vi "Acquisition Core.vi"(6 "Acquired z-plane index":i32, 8 "error in":errorcluster, 9 "AOL_Globals":T5={"Imaging Protocol"=enum."AOL Z-Stack", "Number of POI"=0, "Number of Miniscans"=0, "Number of Trials"=0, "Number of Cycles "=0, "# Averaged Frames"=0, "Laser power (%)"=0, "Pockels"=0.0, "Acquisition Length (sec)"=0.0, "Fill time (us)"=0.0, "POI Dwell time (us)"=0.0, "Miniscan Dwell time per pixel (us)"=0.0, "PMT 1"=0.0, "PMT 2"=0.0, "Back Apperture"=200.0, "Frame Size"=0, "Center Frequency"=0.0, "Field of View"=0.0, "DwellTime (us)"=0.0, "Wavelength (nm)"=0.0, "Zoom"=0.0, "AOL Z"=0.0, "AOL Mode"=enum."Raster", "GridXY"=0.0, "GridZ"=0.0, "TriggerPeriod (sec)"=0.0, "Number of Pixels in Miniscan"=0, "Experiment folder path"=path "", "X centre"=0.0, "Y centre"=0.0, "Angle (degrees)"=0.0, "Plane Mode"=0, "Threshold"=[], "Regenerate Chirps"=FALSE, "Rectangle ROI length (pixels)"=0, "Rectangle ROI height (pixels)"=0, "AOD fill"=0, "Samples Wait after Trigger"=0, "StartUp Delay"=0, "Slip Cycle"=163840, "Add Cycle"=FALSE} {"Plane Mode" items=["XY Plane"]; "Frame Size" items=["100X100"=100, "128X128"=128, "200X200"=200, "256X256"=256, "512X512"=512, "1024x1024"=1024, "2048x2048"=2048]; "Back Apperture" format="%#.6g"; "Pockels" format="%#.6g"; "PMT 2" format="%#.6g"; "PMT 1" format="%#.6g"; "Angle (degrees)" format="%#.6g"; "POI Dwell time (us)" format="%#.6g"}, 11 "Logging queue in":T8) -> (0 "error out":errorcluster, 1 "Logging queue element":T1={"Imaging Protocol"=enum."Live Imaging", "Number of Trials"=0, "Frame Size"=512, "# Averaged frames"=0, "Dwell time (us)"=0.0, "Index of Z-plane"=0, "Timelapse?"=FALSE, "Logging process is active"=FALSE, "Speed logging enabled"=FALSE, "tdms file ref"=refnum, "path"=path "", "Trial Number"=0, "Expected # points acquired"=FALSE, "Manually stopped"=FALSE, "Ch0 data"=[], "Ch1 data"=[], "Last trial"=FALSE, "Points acquired"={"Ch0 last trial"=0, "Ch1 last trial"=0, "All trials"=0}} {"Frame Size" items=["100X100"=100, "128X128"=128, "200X200"=200, "256X256"=256, "512X512"=512, "1024x1024"=1024, "2048x2048"=2048]; "Dwell time (us)" format="%#.6g"})   [LabVIEW 2013]
uses:
  Typedefs/Data queue ref.ctl
  Typedefs/Logging queue element.ctl
  Typedefs/Imaging Protocols enum.ctl
  Typedefs/Frame Size.ctl
  Typedefs/Acquired points count.ctl
  Typedefs/Controls/AOL_Globals.ctl
  Typedefs/AOL modes.ctl
  Typedefs/Plane Mode.ctl
  Typedefs/HW config states enum.ctl
  Video Rec Signaling/typedefs/Functions enum.ctl
  Global Variables/General Globals.vi
panel:
  out "subVI exec time":u32
  out "VI exec time":u32
  out "Elements Remaining in FIFO":u32
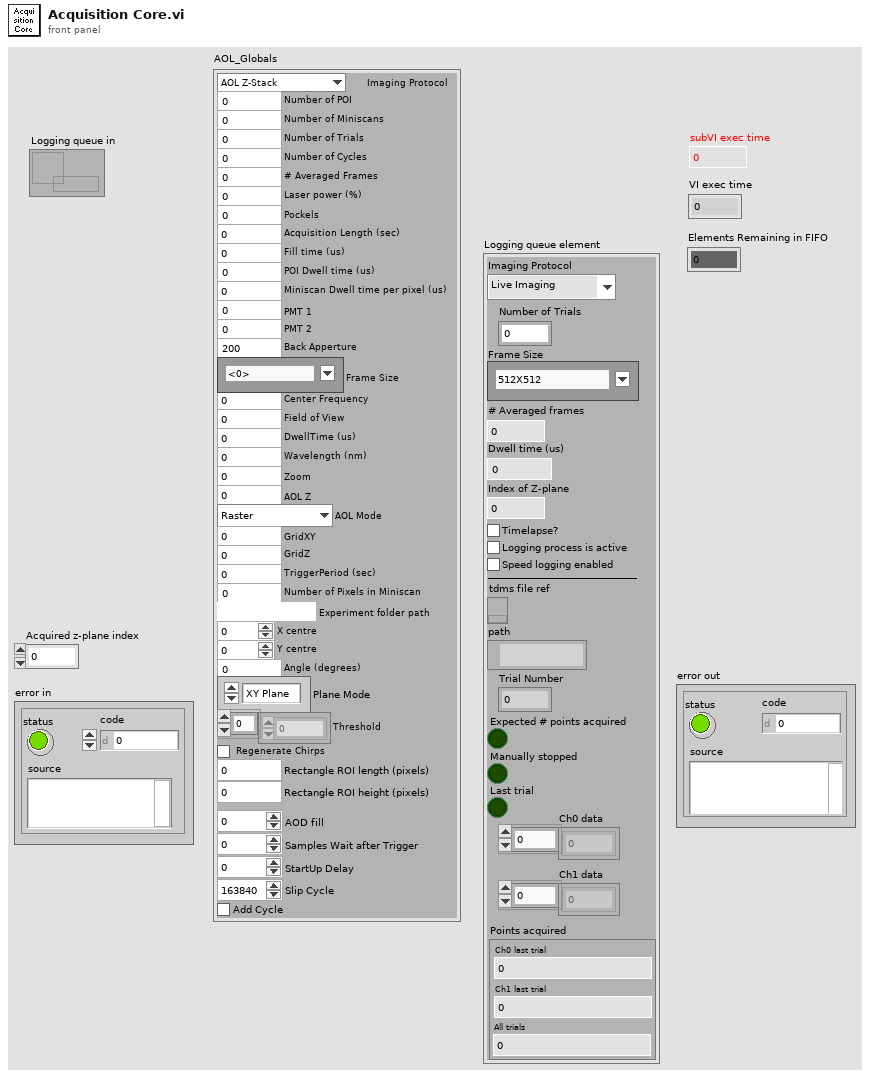
[diagram p1: front panel]
types:
  T1 = typedef "Logging queue element.ctl" = cluster{"Imaging Protocol":T2, "Number of Trials":u16, "Frame Size":T3, "# Averaged frames":u16, "Dwell time (us)":dbl, "Index of Z-plane":i32, "Timelapse?":bool, "Logging process is active":bool, "Speed logging enabled":bool, "tdms file ref":refnum<k34>, "path":path, "Trial Number":i32, "Expected # points acquired":bool, "Manually stopped":bool, "Ch0 data":u32[], "Ch1 data":u32[], "Last trial":bool, "Points acquired":T4}
  T2 = typedef "Imaging Protocols enum.ctl" = enum16{"AOL Z-Stack", "Motor Z Stack", "Functional Acquisition", "Single Plane Acquisition", "Volume Acquisition", "Live Imaging", "Live Plane Imaging", "Live Volume Imaging"}
  T3 = typedef "Frame Size.ctl" = u16
  T4 = typedef "Acquired points count.ctl" = cluster{"Ch0 last trial":u64, "Ch1 last trial":u64, "All trials":u64}
  T5 = typedef "AOL_Globals.ctl" = cluster{"Imaging Protocol":T2, "Number of POI":u16, "Number of Miniscans":u16, "Number of Trials":u16, "Number of Cycles ":u64, "# Averaged Frames":u16, "Laser power (%)":u8, "Pockels":dbl, "Acquisition Length (sec)":dbl, "Fill time (us)":dbl, "POI Dwell time (us)":dbl, "Miniscan Dwell time per pixel (us)":dbl, "PMT 1":dbl, "PMT 2":dbl, "Back Apperture":dbl, "Frame Size":T3, "Center Frequency":dbl, "Field of View":dbl, "DwellTime (us)":dbl, "Wavelength (nm)":dbl, "Zoom":dbl, "AOL Z":dbl, "AOL Mode":T6, "GridXY":dbl, "GridZ":dbl, "TriggerPeriod (sec)":dbl, "Number of Pixels in Miniscan":u16, "Experiment folder path":path, "X centre":dbl, "Y centre":dbl, "Angle (degrees)":dbl, "Plane Mode":T7, "Threshold":u16[], "Regenerate Chirps":bool, "Rectangle ROI length (pixels)":u16, "Rectangle ROI height (pixels)":u16, "AOD fill":u16, "Samples Wait after Trigger":u16, "StartUp Delay":i32, "Slip Cycle":u32, "Add Cycle":bool}
  T6 = typedef "AOL modes.ctl" = enum16{"Raster", "Structural", "Pointing", "Mini Scan", "Alignment"}
  T7 = typedef "Plane Mode.ctl" = u16
  T8 = typedef "Data queue ref.ctl" = refnum<queue>
  T9 = typedef "HW config states enum.ctl" = enum16{"Load from file", "Save to file", "Write all", "Read all", "Write XY stage settings", "Write DAQ FPGA settings", "Write Control FPGA settings", "Write Phys Channels", "Clear", "Compare from file"}
  T10 = typedef "Functions enum.ctl" = enum16{"Create", "Start", "Write", "Stop", "Clear"}
  T11 = typedef "Sys Configuration.ctl" = cluster{"XY Stage":T12, "DAQ FPGA":T13, "Control system":T17, "Encoder":T18, "DAQmx Chan":T19, "Computer MAC address":string, "Cam VidRec":T20, "Externalise Triggers":bool, "Laser wavelength (nm)":dbl}
  T12 = typedef "XY Stage config cluster.ctl" = cluster{"COM port":refnum<visa-resource-name>, "XY stage available":bool}
  T13 = typedef "DAQ FPGA config cluster.ctl" = cluster{"Ref":T14, "Target":T15, "Clock Freq (MHz) ":dbl, "input card type":T16, "Samples Wait after Trigger":u16, "AOD fill":u16, "StartupDelay":i32, "Slip Cycle (clock cycles)":u32, "Add Cycle":bool}
  T14 = typedef "FPGA Ref.ctl" = refnum<k20>
  T15 = typedef "nirio_resource_hc.ctl" = tag
  T16 = typedef "FPGA input type AC-DC.ctl" = enum16{"AC Card", "DC Card"}
  T17 = typedef "CTRL system config cluster.ctl" = cluster{"Ethernet opened":bool, "Ethernet Port":u32, "Ctrl FPGA available":bool, "Ctrl FPGA Clock (MHz)":dbl, "Ctrl system MAC address":string, "Control system.Network adapter name":string, "AOD 1 Amplitude":i16, "AOD 2 Amplitude":i16, "AOD 3 Amplitude":i16, "AOD 4 Amplitude":i16, "Data Time Interval (ns)":dbl, "T0 (ns)":dbl, "Ta (ns)":dbl}
  T18 = typedef "Encoder config cluster.ctl" = cluster{"IP address":string, "Port":u16, "Encoder available":bool, "Wheel radius (cm)":dbl}
  T19 = typedef "DAQmx physical channels cluster.ctl" = cluster{"Pockels AO":tag, "Hard shutter AO":tag, "PMT AOs":tag, "Power meter AI":tag}
  T20 = typedef "Cam VidRec HW config setup cluster.ctl" = cluster{"DO flag-Video record":tag, "DO flag-Trial start":tag, "VidRec available":bool}
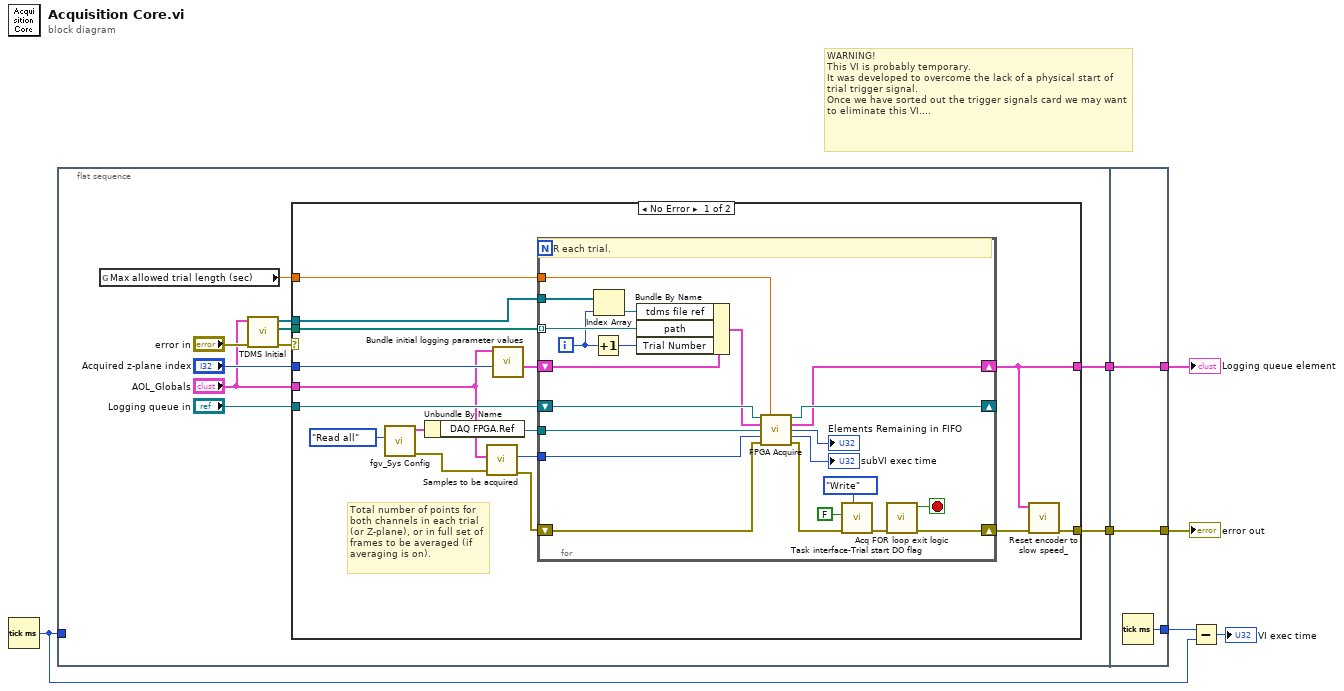
[diagram p0: block diagram]
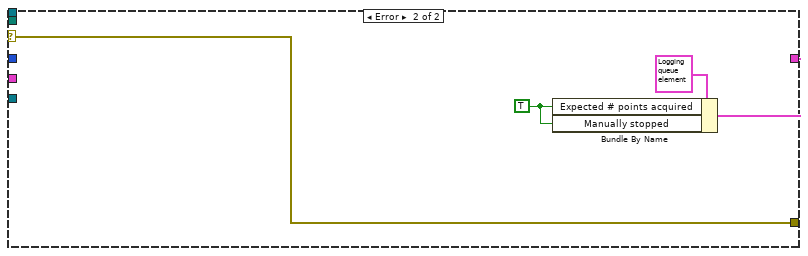
[diagram p2: hidden frame]
diagram:
  # "WARNING!\nThis VI is probably temporary.\nIt was developed to overcome the lack of a physical start of trial trigger signal.\nOnce we have sorted out the trigger signals card we may want to eliminate this VI...."
  n1 = Tick Count (ms)() -> (millisecond timer value=w1:u32)
  n2 = flat-sequence {
    tunnel: w1 -> [_]
    tunnel: [w13] -> w5
    tunnel: [w8] -> w2
    tunnel: [w62] -> w7
    tunnel: [w61] -> w4
    tunnel: w5 -> [w61]
    tunnel: [w60] -> w3
    tunnel: w2 -> [w60]
    frame #0 {
      n3 = global read "General Globals.vi" "Max allowed trial length (sec)"() -> (w9:dbl)
      n4 = call "TDMS Initial.vi"("error in"="error in", "AOL_Globals"="AOL_Globals") -> ("error IO"=w16:errorcluster, "TDMS file paths OR experiment folder path"=w14:path[], "Functional imaging TDMS file references"=w15:refnum<k34>[])  [unwired: 7 in]
      n5 = case shown="No Error" w16 {
        selector: w16 -> [_ w56]
        tunnel: "Logging queue in" -> [w33 _]
        tunnel: w15 -> [w32 _]
        tunnel: w14 -> [w31 _]
        tunnel: [w26 w56] -> w8
        tunnel: "AOL_Globals" -> [w20 _]
        tunnel: "Acquired z-plane index" -> [w28 _]
        tunnel: [w25 w57] -> w13
        tunnel: w9 -> [w27 _]
        frame No Error {
          # "Total number of points for both channels in each trial (or Z-plane), or in full set of frames to be averaged (if averaging is on)."
          n6 = call "fgv_Sys Config.vi"("Function"=HW_config_states_enum."Read all") -> ("error out"=w19:errorcluster, "System Config out"=w23:T11)  [unwired: 9 in]
          n7 = Unbundle By Name(w23) -> ("DAQ FPGA.Ref"=w21:T14)
          n8 = call "Samples to be acquired.vi"("error in (no error)"=w19, "AOL_Globals"=w20) -> ("error out"=w18:errorcluster, "Number of samples to be acquired (points in frame x Ch. x Av.)"=w29:u64)  [unwired: 8 in]
          n9 = call "Bundle initial logging parameter values.vi"("Index of Z plane"=w28, "AOL_Globals IN"=w20) -> ("Logging queue element"=w30:T1)  [unwired: 9 in]
          n10 = for {
            shift-right: [w46] -> _
            shift-left: w33 -> [w51]
            tunnel: w29 -> [w50]
            tunnel: w32 -> [w54]
            tunnel: w31 -> [w49] mode=indexing
            shift-right: [w34] -> w24
            shift-left: w18 -> [w44]
            tunnel: w21 -> [w47]
            tunnel: w27 -> [w41]
            shift-right: [w37] -> w25
            shift-left: w30 -> [w48]
            i -> [w40]
            stop <- w52 stop-if-true
            # "FOR each trial."
            n11 = Increment(x=w40) -> (x+1=w55:i32)
            n12 = Index Array(array=w54, index=w40) -> (element=w53:refnum<k34>)
            n13 = Bundle By Name(cluster=w48, "tdms file ref"=w53, "path"=w49, "Trial Number"=w55) -> (w45:T1)
            n14 = call "FPGA Acquire.vi"("Logging queue in"=w51, "Max allowed trial length (sec)"=w41, "Logging queue element"=w45, "FPGA Ref"=w47, "Target number of points"=w50, "error in (no error)"=w44) -> ("Logging queue out"=w46:T8, "Logging queue element"=w37:T1, "Elements Remaining"=→"Elements Remaining in FIFO":u32, "VI exec time"=→"subVI exec time":u32, "error out"=w36:errorcluster)  [unwired: 5 in]
            n15 = call "Task interface-Trial start DO flag.vi"("Function"=Functions_enum."Write", "error in"=w36, "DO value"=FALSE) -> ("error out"=w35:errorcluster)  [unwired: 8 in]
            n16 = call "Acq FOR loop exit logic.vi"("error in (no error)"=w35) -> ("error out (dupl)"=w34:errorcluster, "Stop acquisition FOR loop"=w52:bool)  [unwired: 9 in]
          }
          n17 = call "Reset encoder to slow speed_.vi"("error in (no error)"=w24, "Logging queue element"=w25) -> ("error out"=w26:errorcluster)  [unwired: 9 in]
        }
        frame Error {
          w59 = TRUE ("Manually stopped")
          n18 = Bundle By Name(cluster=T1 {"Imaging Protocol"=enum."AOL Z-Stack", "Number of Trials"=0, "Frame Size"=0, "# Averaged frames"=0, "Dwell time (us)"=0.0, "Index of Z-plane"=0, "Timelapse?"=FALSE, "Logging process is active"=FALSE, "Speed logging enabled"=FALSE, "tdms file ref"=refnum, "path"=path "", "Trial Number"=0, "Expected # points acquired"=FALSE, "Manually stopped"=FALSE, "Ch0 data"=[], "Ch1 data"=[], "Last trial"=FALSE, "Points acquired"={"Ch0 last trial"=0, "Ch1 last trial"=0, "All trials"=0}} ("Logging queue element"), "Expected # points acquired"=w59, "Manually stopped"=w59) -> (w57:T1)
        }
      }
    }
    frame #1 {
      n19 = Tick Count (ms)() -> (millisecond timer value=w62:u32)
    }
  }
  n20 = Subtract(x=w7, y=w1) -> (x-y=→"VI exec time":u32)
  "Logging queue element" <- w4
  "error out" <- w3
